vi "PH_HamamatsuCamera.PC set ROI.vi"(0 "VI in":refnum<vi>, 2 "Horizontal Offset":T1, 5 "error in (no error)":errorcluster) -> (14 "VI out":refnum<vi>, 19 "error out":errorcluster)   [LabVIEW 2014, in "PH_HamamatsuCamera.lvlib"]
uses:
  PH_HamamatsuCamera.lvlib
  PH_HamamatsuCamera.ROI.ctl
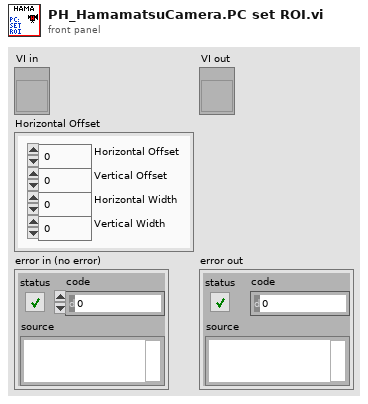
[diagram p1: front panel]
types:
  T1 = typedef "PH_HamamatsuCamera.lvlib/PH_HamamatsuCamera.ROI.ctl" = cluster{"Horizontal Offset":i32, "Vertical Offset":i32, "Horizontal Width":i32, "Vertical Width":i32}
  T2 = typedef "PH_HamamatsuCamera.lvlib/PH_HamamatsuCamera.i attribute.ctl" = cluster{"Gui Refs":cluster{"Camera Details":refnum<vi>, "ROI":refnum<vi>, "Set ROI to Maximum":refnum<vi>, "Trigger Parameters":refnum<vi>, "Brightness":refnum<vi>, "Shutter":refnum<vi>, "Gain":refnum<vi>, "Trigger Timeout":refnum<vi>, "Trigger Polarity":refnum<vi>, "Trigger Mode":refnum<vi>, "Parameters":refnum<vi>, "Set Cam Parameter":refnum<vi>, "Parameter to set":refnum<vi>, "Value to set":refnum<vi>}, "Cam":cluster{"Handle":i32, "Details":cluster{"Model":string, "Camera ID":string, "Firmware":string}, "Buffer Info":cluster{"height":u32, "width":u32, "datatype":u32}}, "H Offset":cluster{"Value":i32, "Minimum":i32, "Maximum":i32, "Increment":i32}, "V Offset":cluster{"Value":i32, "Minimum":i32, "Maximum":i32, "Increment":i32}, "H Width":cluster{"Value":i32, "Minimum":i32, "Maximum":i32, "Increment":i32}, "V Width":cluster{"Value":i32, "Minimum":i32, "Maximum":i32, "Increment":i32}, "Trigger Parameters":T3, "Trigger Timeout":u32, "Parameters":T4[], "Indicees Cam Parameters":cluster{"Brightness":i32, "Shutter":i32, "Gain":i32}, "Wanted Values":cluster{"Trigger Settings":T3[], "ROI":T1[], "Parameter":cluster{"Name":string, "Value":dbl}[]}}
  T3 = typedef "PH_HamamatsuCamera.lvlib/PH_HamamatsuCamera.Trigger Parameter.ctl" = cluster{"Mode":u32, "Polarity":u32, "Times":u32, "Delay":dbl}
  T4 = typedef "PH_HamamatsuCamera.lvlib/PH_HamamatsuCamera.Parameter Set.ctl" = cluster{"Parameter":string, "Value":dbl, "Writable":bool, "Range":cluster{"min":dbl, "max":dbl, "step":dbl}, "Default":dbl, "Value Names":cluster{"Name":string, "Value":dbl}[], "Text Values":bool}
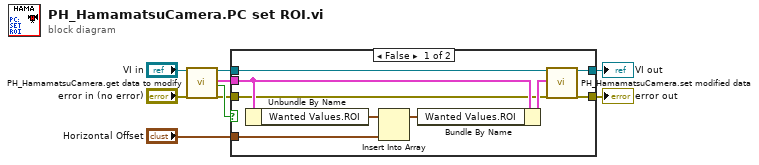
[diagram p0: block diagram]
diagram:
  n1 = call "PH_HamamatsuCamera.get data to modify.vi"("i ref in"="VI in", "error in (no error)"="error in (no error)") -> ("i ref out"=w5:refnum<vi>, "i attribute"=w8:T2, "timed out"=w7:bool, "error out"=w6:errorcluster)  [unwired: 14 in]
  n2 = case shown="False" w7 {
    tunnel: w5 -> [w18 w20]
    tunnel: w6 -> [w11 w19]
    tunnel: [w13 w20] -> w1
    tunnel: [w12 w19] -> w2
    tunnel: w8 -> [w16 _]
    tunnel: "Horizontal Offset" -> [w10 _]
    frame False {
      n3 = Unbundle By Name(w16) -> ("Wanted Values.ROI"=w15:T1[])
      n4 = Insert Into Array(array=w15, new element=w10) -> (w14:T1[])  [unwired: 1 in]
      n5 = Bundle By Name(cluster=w16, "Wanted Values.ROI"=w14) -> (w17:T2)
      n6 = call "PH_HamamatsuCamera.set modified data.vi"("i ref in"=w18, "i attribute"=w17, "error in (no error)"=w11) -> ("i ref out"=w13:refnum<vi>, "error out"=w12:errorcluster)  [unwired: 15 in]
    }
    frame True {
    }
  }
  "error out" <- w2
  "VI out" <- w1
